vi "Write G08 Clock Params.vi"(8 "error in (no error)":errorcluster, 9 "Trigger Multiplier":u32, 10 "Trigger Divider":u32, 11 "BME_DG_G08 in":refnum<class "BME_DG_G08.lvclass">) -> (0 "error out":errorcluster, 3 "BME_DG_G08 out":refnum<class "BME_DG_G08.lvclass">)   [LabVIEW 2009, in "POLARIS BME DG.lvlib" / "BME_DG_G08.lvclass"]
uses:
  BME_DG_G08.lvclass
  BME_DG_G08.lvclass/BME_DG_G08.ctl
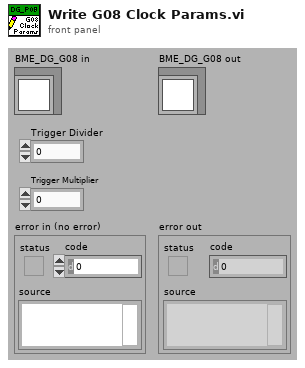
[diagram p1: front panel]
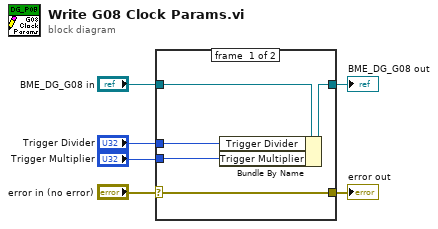
[diagram p0: block diagram]
diagram:
  n1 = case shown="No Error" "error in (no error)" {
    selector: "error in (no error)" -> [w11 w12]
    tunnel: [w11 w12] -> w5
    tunnel: [w9 w13] -> w3
    tunnel: "BME_DG_G08 in" -> [w10 w13]
    tunnel: "Trigger Multiplier" -> [w8 _]
    tunnel: "Trigger Divider" -> [w7 _]
    frame #0 {
      n2 = Bundle By Name(cluster=w10, "Trigger Divider"=w7, "Trigger Multiplier"=w8) -> (w9:refnum<class "BME_DG_G08.lvclass">)
    }
    frame #1 {
    }
  }
  "error out" <- w5
  "BME_DG_G08 out" <- w3
